vi "Read Array Shared Variables.vi"() -> ()   [LabVIEW 2014]
panel:
  in  "Array of Type code":i32[](array[numeric])
  in  "Array of SV Refnums":refnum<k21>[](array[refnum])
  in  "Array of Waveform":waveform(dbl)[](array[waveform])
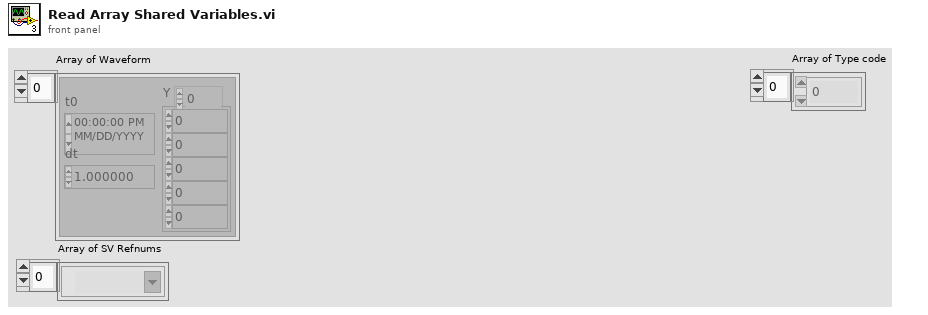
[diagram p1: front panel]
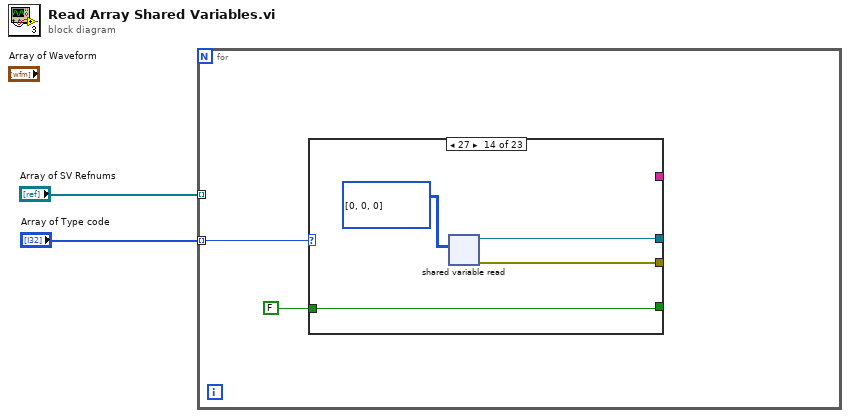
[diagram p0: block diagram]
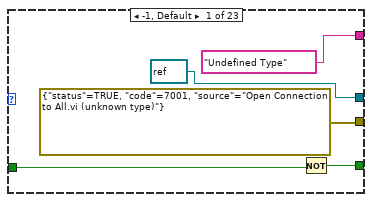
[diagram p2: hidden frame]
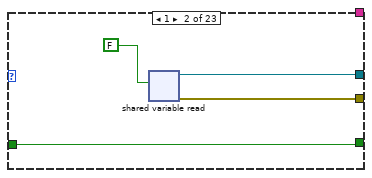
[diagram p3: hidden frame]
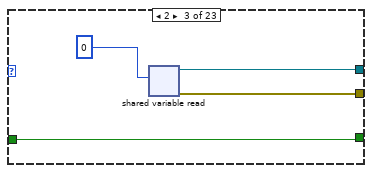
[diagram p4: hidden frame]
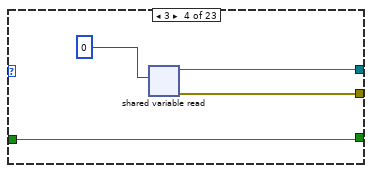
[diagram p5: hidden frame]
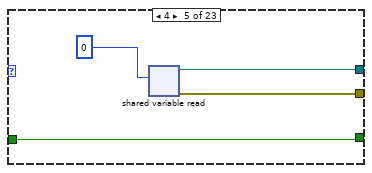
[diagram p6: hidden frame]
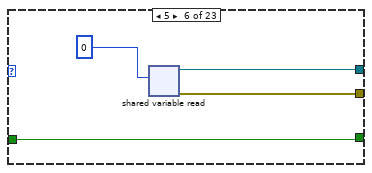
[diagram p7: hidden frame]
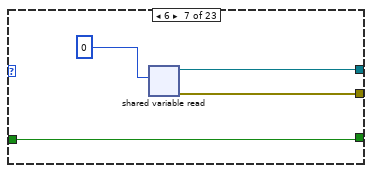
[diagram p8: hidden frame]
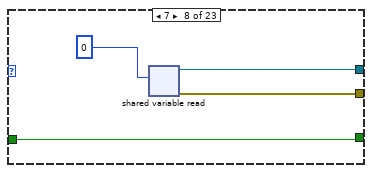
[diagram p9: hidden frame]
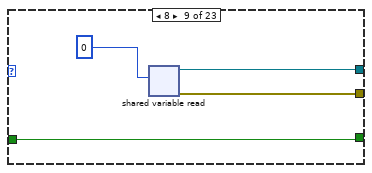
[diagram p10: hidden frame]
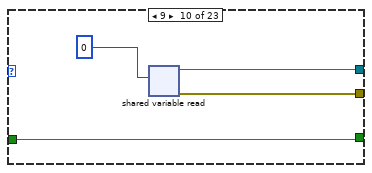
[diagram p11: hidden frame]
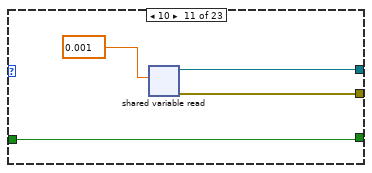
[diagram p12: hidden frame]
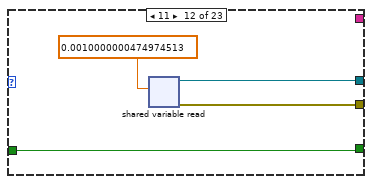
[diagram p13: hidden frame]
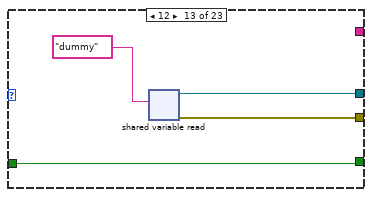
[diagram p14: hidden frame]
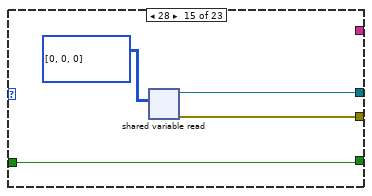
[diagram p15: hidden frame]
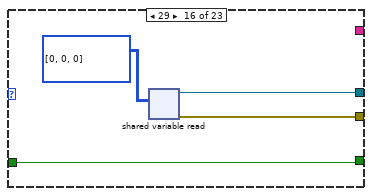
[diagram p16: hidden frame]
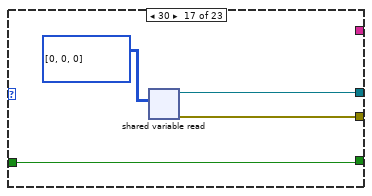
[diagram p17: hidden frame]
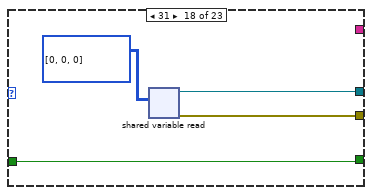
[diagram p18: hidden frame]
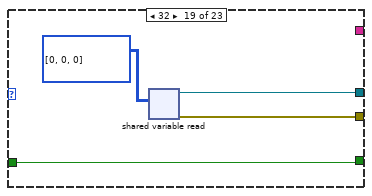
[diagram p19: hidden frame]
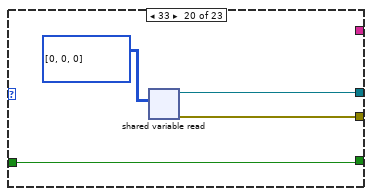
[diagram p20: hidden frame]
diagram:
  n1 = for {
    tunnel: "Array of SV Refnums" -> [_] mode=indexing
    tunnel: "Array of Type code" -> [w4] mode=indexing
    n2 = case shown="27" w4 {
      tunnel: [errorcluster {"status"=TRUE, "code"=7001, "source"="Open Connection to All.vi (unknown type)"} ("error constant") w12 w16 w20 w24 w28 w32 w36 w40 w44 w48 w52 w56 w60 w64 w68 w72 w76 w80 w84 w88 w92 w96] -> _
      tunnel: ["Undefined Type" _ _ _ _ _ _ _ _ _ _ _ _ _ _ _ _ _ _ _ _ _ _] -> _
      tunnel: [w8 w10 w14 w18 w22 w26 w30 w34 w38 w42 w46 w50 w54 w58 w62 w66 w70 w74 w78 w82 w86 w90 w94] -> _
      tunnel: [refnum<k21> refnum w11 w15 w19 w23 w27 w31 w35 w39 w43 w47 w51 w55 w59 w63 w67 w71 w75 w79 w83 w87 w91 w95] -> _
      tunnel: FALSE -> [w5 w10 w14 w18 w22 w26 w30 w34 w38 w42 w46 w50 w54 w58 w62 w66 w70 w74 w78 w82 w86 w90 w94]
      frame -1, Default {
        n3 = Not(x=w5) -> (.not. x?=w8:bool)
      }
      frame 1 {
        n4 = shared-variable-read(FALSE) -> (w11:refnum<k21>, w12:errorcluster)  [unwired: 2 in, 2 out]
      }
      frame 2 {
        n5 = shared-variable-read(i8 0) -> (w15:refnum<k21>, w16:errorcluster)  [unwired: 2 in, 2 out]
      }
      frame 3 {
        n6 = shared-variable-read(i16 0) -> (w19:refnum<k21>, w20:errorcluster)  [unwired: 2 in, 2 out]
      }
      frame 4 {
        n7 = shared-variable-read(0) -> (w23:refnum<k21>, w24:errorcluster)  [unwired: 2 in, 2 out]
      }
      frame 5 {
        n8 = shared-variable-read(i64 0) -> (w27:refnum<k21>, w28:errorcluster)  [unwired: 2 in, 2 out]
      }
      frame 6 {
        n9 = shared-variable-read(u8 0) -> (w31:refnum<k21>, w32:errorcluster)  [unwired: 2 in, 2 out]
      }
      frame 7 {
        n10 = shared-variable-read(u16 0) -> (w35:refnum<k21>, w36:errorcluster)  [unwired: 2 in, 2 out]
      }
      frame 8 {
        n11 = shared-variable-read(u32 0) -> (w39:refnum<k21>, w40:errorcluster)  [unwired: 2 in, 2 out]
      }
      frame 9 {
        n12 = shared-variable-read(u64 0) -> (w43:refnum<k21>, w44:errorcluster)  [unwired: 2 in, 2 out]
      }
      frame 10 {
        n13 = shared-variable-read(0.001) -> (w47:refnum<k21>, w48:errorcluster)  [unwired: 2 in, 2 out]
      }
      frame 11 {
        n14 = shared-variable-read(sgl 0.001) -> (w51:refnum<k21>, w52:errorcluster)  [unwired: 2 in, 2 out]
      }
      frame 12 {
        n15 = shared-variable-read("dummy") -> (w55:refnum<k21>, w56:errorcluster)  [unwired: 2 in, 2 out]
      }
      frame 27 {
        n16 = shared-variable-read(i16[][] [[0, 0, 0]]) -> (w59:refnum<k21>, w60:errorcluster)  [unwired: 2 in, 2 out]
      }
      frame 28 {
        n17 = shared-variable-read(i32[][] [[0, 0, 0]]) -> (w63:refnum<k21>, w64:errorcluster)  [unwired: 2 in, 2 out]
      }
      frame 29 {
        n18 = shared-variable-read(i64[][] [[0, 0, 0]]) -> (w67:refnum<k21>, w68:errorcluster)  [unwired: 2 in, 2 out]
      }
      frame 30 {
        n19 = shared-variable-read(u8[][] [[0, 0, 0]]) -> (w71:refnum<k21>, w72:errorcluster)  [unwired: 2 in, 2 out]
      }
      frame 31 {
        n20 = shared-variable-read(u16[][] [[0, 0, 0]]) -> (w75:refnum<k21>, w76:errorcluster)  [unwired: 2 in, 2 out]
      }
      frame 32 {
        n21 = shared-variable-read(u32[][] [[0, 0, 0]]) -> (w79:refnum<k21>, w80:errorcluster)  [unwired: 2 in, 2 out]
      }
      frame 33 {
        n22 = shared-variable-read(u64[][] [[0, 0, 0]]) -> (w83:refnum<k21>, w84:errorcluster)  [unwired: 2 in, 2 out]
      }
      frame 34 {
        n23 = shared-variable-read(dbl[][] [[0.0, 0.0, 0.0]]) -> (w87:refnum<k21>, w88:errorcluster)  [unwired: 2 in, 2 out]
      }
      frame 35 {
        n24 = shared-variable-read(sgl[][] [[0.0, 0.0, 0.0]]) -> (w91:refnum<k21>, w92:errorcluster)  [unwired: 2 in, 2 out]
      }
      frame 36 {
        n25 = shared-variable-read(string[][] []) -> (w95:refnum<k21>, w96:errorcluster)  [unwired: 2 in, 2 out]
      }
    }
  }
